vi "json token return at.vi"(9 "string index":i32, 10 "token in":i32, 11 "tokens in":T1[](array[typedef])) -> (2 "token out":i32, 3 "tokens out":T1[](array[typedef]))   [LabVIEW 2013]
uses:
  json token.ctl
  json node type.ctl
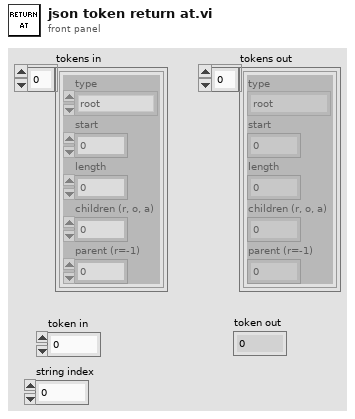
[diagram p1: front panel]
types:
  T1 = typedef "json token.ctl" = cluster{"type":T2, "start":i32, "length":i32, "children (r, o, a)":u16, "parent (r=-1)":i32}
  T2 = typedef "json node type.ctl" = enum16{"root", "object", "array", "number", "string value", "string key", "true", "false", "null"}
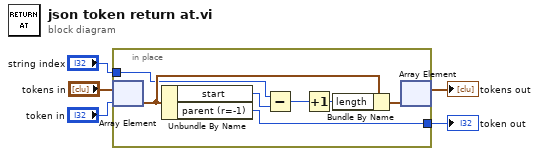
[diagram p0: block diagram]
diagram:
  n1 = in-place {
    in-place-border: [w12] -> w2
    in-place-border: "string index" -> [w8]
    n2 = in-place-array #1("tokens in", "token in") -> (w11:T1)
    n3 = Unbundle By Name(w11) -> ("start"=w7:i32, "parent (r=-1)"=w12:i32)
    n4 = Subtract(x=w8, y=w7) -> (x-y=w9:i32)
    n5 = Increment(x=w9) -> (x+1=w6:i32)
    n6 = Bundle By Name(cluster=w11, "length"=w6) -> (w10:T1)
    n7 = in-place-array #1(w10) -> (→"tokens out":T1[])  [unwired: 1 out]
  }
  "token out" <- w2
